vi "getEnumeratorIntValue.vi"(8 "error in (no error)":errorcluster, 11 "IEnumerationType in":refnum<class "IEnumerationType.lvclass">) -> (0 "error out":errorcluster, 2 "Int Value out":i64, 3 "IEnumerationType out":refnum<class "IEnumerationType.lvclass">)   [LabVIEW 2022 SP3, in "openDAQ.lvlib" / "daqCoreTypes.lvlib" / "IEnumerationType.lvclass"]
uses:
  <instrlib>/openDAQ/Public/Classes/daqCoreTypes/IEnumerationType/IEnumerationType.lvclass
  C:/Program Files (x86)/National Instruments/LabVIEW 2022/instr.lib/openDAQ/Public/Classes/IBaseObject/IBaseObject.lvclass
  <instrlib>/openDAQ/Public/Classes/IBaseObject/IBaseObject.lvclass/IBaseObject.ctl
  <instrlib>/openDAQ/Public/Classes/IBaseObject/Accessor/Read reference.vi
  <instrlib>/openDAQ/Public/Classes/IBaseObject/Accessor/Write reference.vi
  <instrlib>/openDAQ/Binaries/Windows/x86/copendaq32.dll
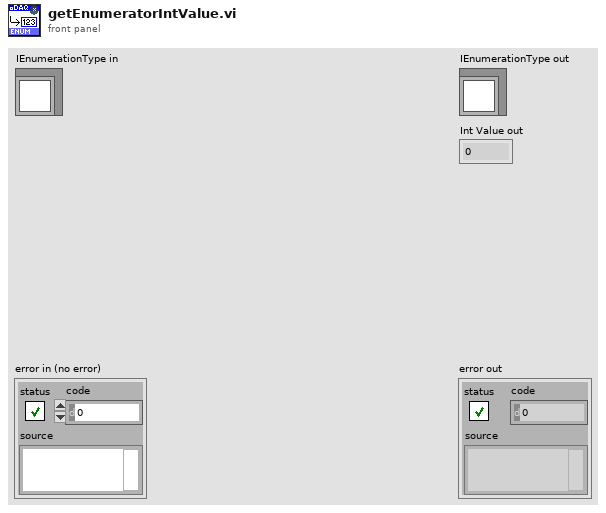
[diagram p1: front panel]
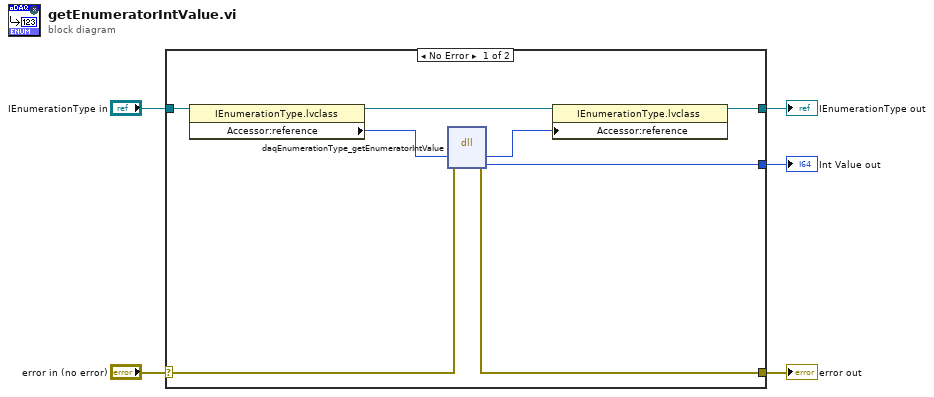
[diagram p0: block diagram]
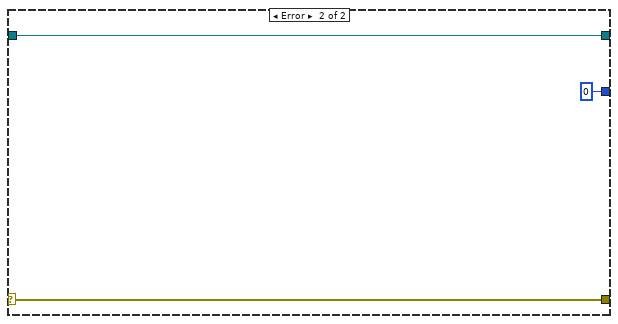
[diagram p2: hidden frame]
diagram:
  n1 = case shown="No Error" "error in (no error)" {
    selector: "error in (no error)" -> [w7 w16]
    tunnel: [w8 w16] -> w4
    tunnel: [w11 w15] -> w2
    tunnel: "IEnumerationType in" -> [w13 w15]
    tunnel: [w6 i64 0 ("intValue")] -> w1
    frame No Error {
      n2 = property class="IEnumerationType.lvclass"(reference=w13) -> (reference out=w12:refnum<class "IEnumerationType.lvclass">, "Accessor:reference"=w10:i64)  [unwired: 1 in, 1 out]
      n3 = dll-call lib="C:/Program Files (x86)/National Instruments/LabVIEW 2022/instr.lib/openDAQ/Binaries/Windows/x86/copendaq*.*" fn="daqEnumerationType_getEnumeratorIntValue"(error in=w7, "enumerationType"=w10) -> (error out=w8:errorcluster, "enumerationType"=w9:i64, "intValue"=w6:i64)  [unwired: 4 in, 1 out]
      n4 = property class="IEnumerationType.lvclass"(reference=w12, "Accessor:reference"=w9) -> (reference out=w11:refnum<class "IEnumerationType.lvclass">)  [unwired: 1 in, 1 out]
    }
    frame Error {
    }
  }
  "error out" <- w4
  "IEnumerationType out" <- w2
  "Int Value out" <- w1
